vi "NI 5752 Finite Acquisition Multiple Channels (Host).vi"() -> ()   [LabVIEW 2014]
uses:
  <vilib>/rvi/interface/nirviOpenFPGA/nirviOpenFPGA.xnode
  <vilib>/rvi/interface/nirviReadWriteControl/nirviReadWriteControl.xnode
  <vilib>/rvi/interface/nirviCloseFPGA/nirviCloseFPGA.xnode
  <vilib>/rvi/interface/nirviMethod/nirviMethod.xnode
  Program Files (x86)/National Instruments/LabVIEW 2014/examples/FlexRIO/IO Modules/NI 5752/FiniteAcqMultipleChannels/NI 5752 Finite Acquisition Multiple Channels (FPGA).vi
  FPGA Bitfiles/NI5752Fini_PXI-7952R.lvbitx
  <vilib>/LabVIEW Targets/FPGA/FlexRIO/CustomFPGAMethods/79XXR_Method_IOModuleStatusImpl.vi
  NiFpgaLv.dll
  <vilib>/Utility/error.llb/Error Cluster From Error Code.vi
  <vilib>/rvi/errors/niLvFpgaAdjustHostInterfaceError.vi
  <vilib>/FPGAPlugInAG/PXI-7952R/niLvFpga_ReadFifo_PXI-7952R.vi
  <vilib>/rvi/errors/niLvFpgaMergeErrorWithErrorCode.vi
  <vilib>/FPGAPlugInAG/PXI-7952R/niLvFpga_Close_PXI-7952R.vi
  <vilib>/FPGAPlugInAG/PXI-7952R/niLvFpga_Open_PXI-7952R.vi
  <vilib>/userdefined/High Color/nirio_resource_hc.ctl
panel:
  in  "RIO Device":T1="RIO0"
  in  "stop":bool
  in  "ADC D":bool
  in  "ADC C":bool
  in  "ADC B":bool
  in  "ADC A":bool=TRUE
  out "error out":errorcluster
  in  "Tab Control":enum32{"ADC A", " ADC B", "ADC C", "ADC D"}(tab)
  out "ADC A Graph":dbl[][](graph)
  out "ADC B Graph":dbl[][](graph)
  out "ADC C Graph":dbl[][](graph)
  out "ADC D Graph":dbl[][](graph)
  # "ADCs to Acquire"
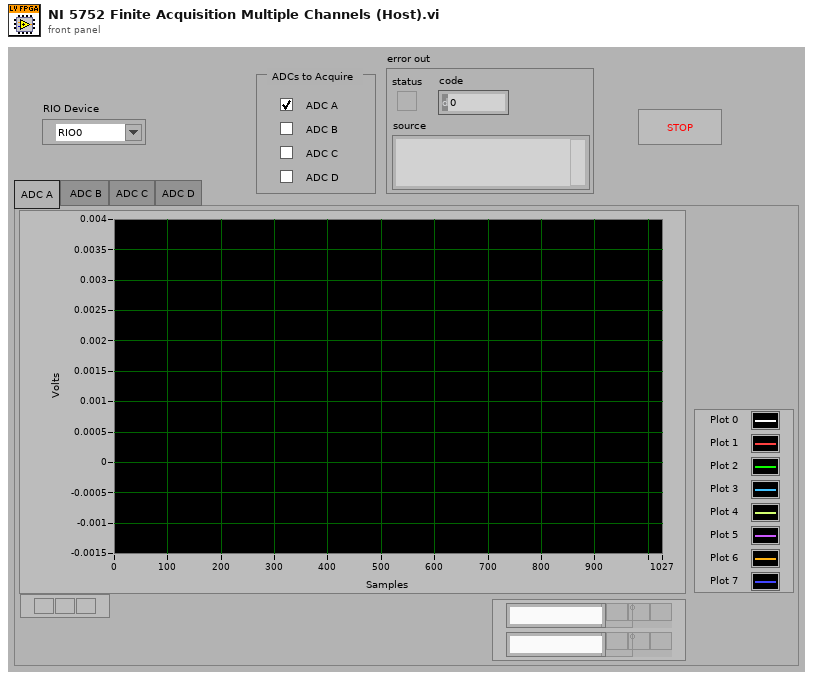
[diagram p1: front panel]
types:
  T1 = typedef "nirio_resource_hc.ctl" = tag
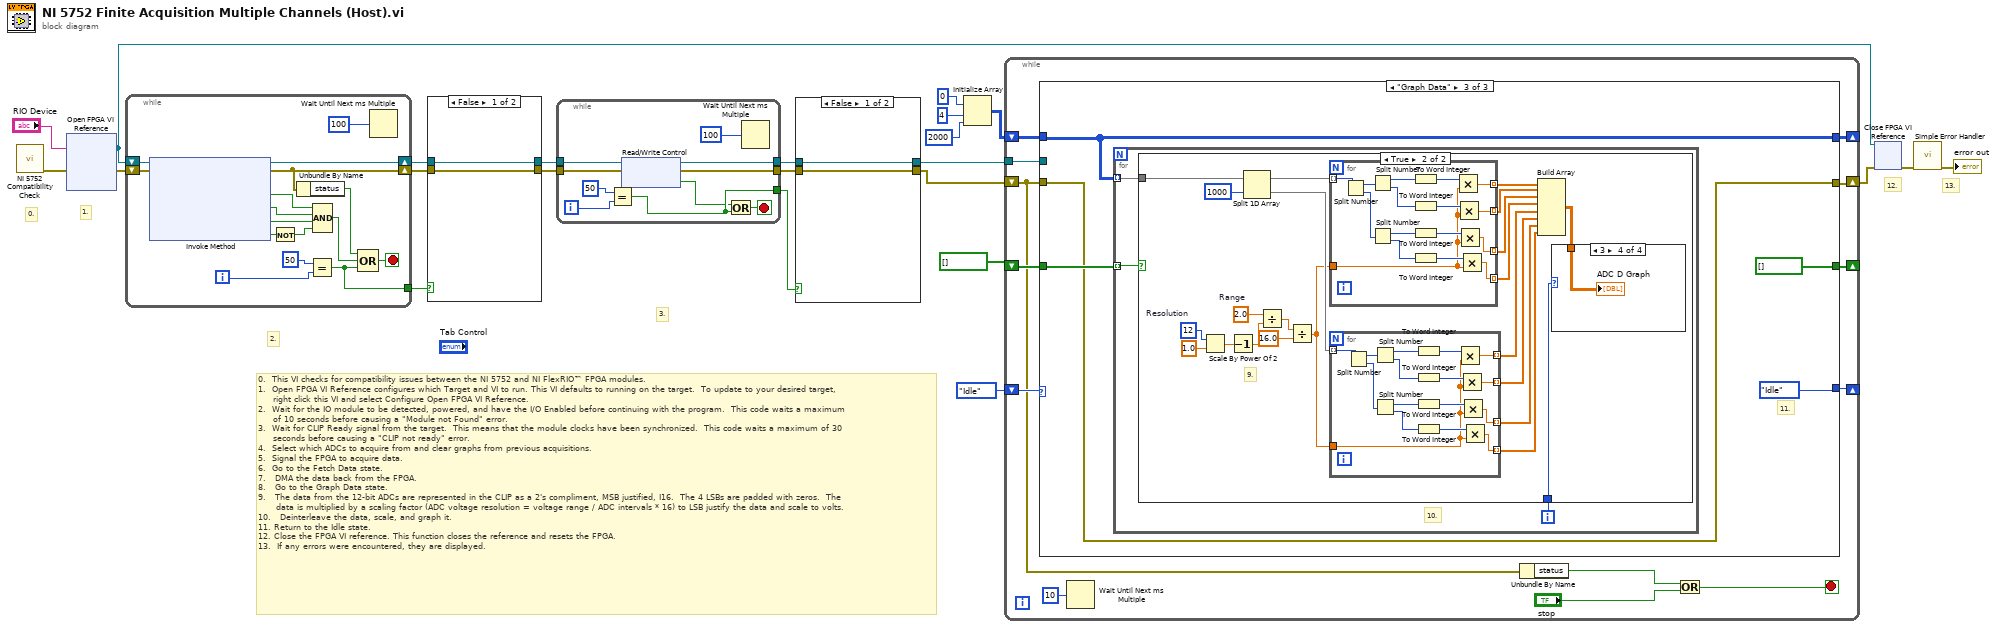
[diagram p0: block diagram]
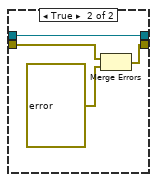
[diagram p2: hidden frame]
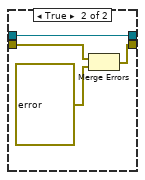
[diagram p3: hidden frame]
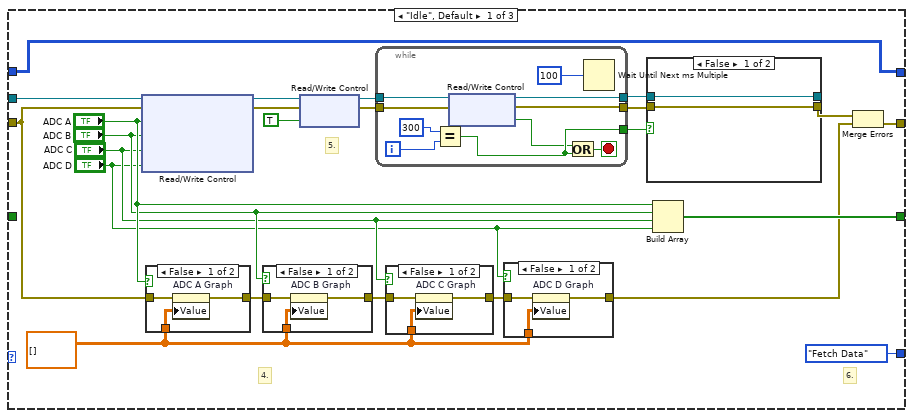
[diagram p4: hidden frame]
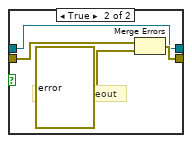
[diagram p5: hidden frame]
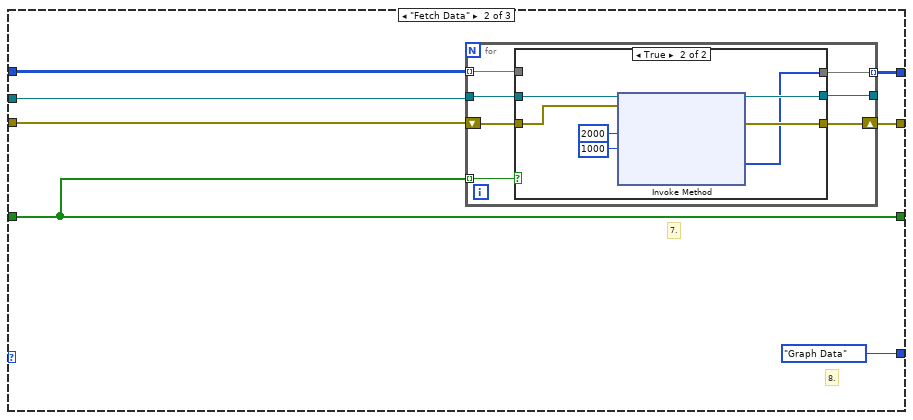
[diagram p10: hidden frame]
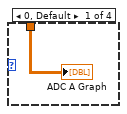
[diagram p13: hidden frame]
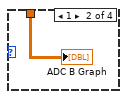
[diagram p14: hidden frame]
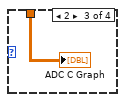
[diagram p15: hidden frame]
diagram:
  # "0."
  # "3."
  # "13."
  # "12."
  # "2."
  # "0.  This VI checks for compatibility issues between the NI 5752 and NI FlexRIO™ FPGA modules. \n1.  Open FPGA VI Reference configures which Target and VI to run. This VI defaults to running on the target.  To update to your desired target, \n     right click this VI and select Configure Open FPGA VI Reference.\n2.  Wait for the IO module to be detected, powered, and have the I/O Enabled before continuing with the program.  This code waits a maximum \n     of 10 seconds before causing a \"Module not Found\" error.\n3.  Wait for CLIP Ready signal from the target.  This means that the module clocks have been synchronized.  This code waits a maximum of 30 \n     seconds before causing a \"CLIP not ready\" error.\n4.  Select which ADCs to acquire from and clear graphs from previous acquisitions.\n5.  Signal the FPGA to acquire data.\n6.  Go to the Fetch Data state.\n7.   DMA the data back from the FPGA.\n8.   Go to the Graph Data state.\n9.   The data from the 12-bit ADCs are represented in the CLIP as a 2's compliment, MSB justified, I16.  The 4 LSBs are padded with zeros.  The \n      data is multiplied by a scaling factor (ADC voltage resolution = voltage range / ADC intervals * 16) to LSB justify the data and scale to volts.\n10.   Deinterleave the data, scale, and graph it.\n11. Return to the Idle state.\n12. Close the FPGA VI reference. This function closes the reference and resets the FPGA.\n13.  If any errors were encountered, they are displayed."
  # "1."
  n1 = call "NI 5752 Compatibility Check.vi"() -> ("error out"=w1:errorcluster)  [unwired: 2 in, 9 out]
  n2 = xnode "Open FPGA VI Reference"("error in"=w1, "resource name"="RIO Device") -> ("FPGA VI Reference Out"=w13:refnum<k20>, "error out"=w14:errorcluster)
  n3 = while {
    shift-right: [w30] -> w12
    shift-left: w14 -> [w38]
    shift-right: [w37] -> w10
    shift-left: w13 -> [w39]
    tunnel: [w26] -> w11
    i -> [w32]
    stop <- w27 stop-if-true
    n4 = xnode "Invoke Method"("FPGA VI Reference In"=w39, "error in"=w38) -> ("FPGA VI Reference Out"=w37:refnum<k20>, "error out"=w30:errorcluster, "IO Module Present?"=w36:bool, "Power Enabled?"=w35:bool, "IO Enabled?"=w34:bool, "IO Module Mismatch?"=w25:bool)
    n5 = Not(x=w25) -> (.not. x?=w24:bool)
    n6 = Unbundle By Name(w30) -> ("status"=w29:bool)
    n7 = Equal?(x=50, y=w32) -> (x = y?=w26:bool)
    n8 = Compound Arithmetic op=AND(w36, w35, w34, w24) -> (w28:bool)
    n9 = Compound Arithmetic op=OR(w29, w28, w26) -> (w27:bool)
    n10 = Wait Until Next ms Multiple(millisecond multiple=u32 100) -> ()  [unwired: 1 out]
  }
  n11 = case shown="False" w11 {
    tunnel: w12 -> [w40 w44]
    tunnel: [w40 w43] -> w8
    tunnel: w10 -> [w41 w42]
    tunnel: [w41 w42] -> w9
    frame False {
    }
    frame True {
      n12 = Merge Errors(w44, errorcluster {"status"=TRUE, "code"=-1, "source"="The IO Module was not present, powered, or the IO were not enabled.  Verify the NI 5752 is securly connected and try again."} ("error in")) -> (w43:errorcluster)
    }
  }
  n13 = while {
    tunnel: w9 -> [w55]
    tunnel: [w51] -> w7
    tunnel: [w50] -> w6
    tunnel: [w48] -> w3
    tunnel: w8 -> [w46]
    i -> [w53]
    stop <- w49 stop-if-true
    n14 = Equal?(x=50, y=w53) -> (x = y?=w48:bool)
    n15 = xnode "Read/Write Control"("FPGA VI Reference In"=w55, "error in"=w46) -> ("FPGA VI Reference Out"=w51:refnum<k20>, "error out"=w50:errorcluster, "Init Done"=w47:bool)
    n16 = Or(x=w47, y=w48) -> (x .or. y?=w49:bool)
    n17 = Wait Until Next ms Multiple(millisecond multiple=u32 100) -> ()  [unwired: 1 out]
  }
  n18 = case shown="False" w3 {
    tunnel: w6 -> [w56 w60]
    tunnel: [w56 w59] -> w4
    tunnel: w7 -> [w57 w58]
    tunnel: [w57 w58] -> w5
    frame False {
    }
    frame True {
      n19 = Merge Errors(w60, errorcluster {"status"=TRUE, "code"=-1, "source"="The IO Module CLIP was not ready. If you are using any external clocks, make sure they are connected and within the supported specifications."} ("error in")) -> (w59:errorcluster)
    }
  }
  n20 = Initialize Array(u64 0, 4 ("dimension size"), 2000 ("dimension size")) -> (w20:u64[][])
  n21 = while {
    shift-right: [w73] -> _
    shift-left: enum16{"Idle", "Graph Data", "Fetch Data"}."Idle" -> [w74]
    tunnel: w5 -> [w66]
    shift-right: [w71] -> _
    shift-left: w20 -> [w72]
    shift-right: [w69] -> _
    shift-left: bool[] [] -> [w68]
    shift-right: [w67] -> w16
    shift-left: w4 -> [w65]
    stop <- w62 stop-if-true
    n22 = case shown="\"Graph Data\"" w74 {
      tunnel: w66 -> [w98 w131 _]
      tunnel: w65 -> [w97 w132 w155]
      tunnel: [w96 w133 w155] -> w67
      tunnel: [enum16{"Idle", "Graph Data", "Fetch Data"}."Fetch Data" enum16{"Idle", "Graph Data", "Fetch Data"}."Graph Data" enum16{"Idle", "Graph Data", "Fetch Data"}."Idle"] -> w73
      tunnel: w72 -> [w94 w136 w156]
      tunnel: [w94 w134 w156] -> w71
      tunnel: [w93 w135 bool[] []] -> w69
      tunnel: w68 -> [_ w135 w157]
      frame "Idle", Default {
        w88 = dbl[][] [] ("ADC A Graph")
        # "6."
        # "5."
        # "4."
        n23 = xnode "Read/Write Control"("FPGA VI Reference In"=w98, "error in"=w97, "ADC A Requested"="ADC A", "ADC B Requested"="ADC B", "ADC C Requested"="ADC C", "ADC D Requested"="ADC D") -> ("FPGA VI Reference Out"=w92:refnum<k20>, "error out"=w89:errorcluster)
        n24 = case shown="False" "ADC A" {
          tunnel: w97 -> [w129 w130]
          tunnel: w88 -> [w128 _]
          tunnel: [w127 w130] -> w87
          frame False {
            n25 = property on="ADC A Graph" class="WFGraph (strict)"(error in=w129, "Value"=w128) -> (error out=w127:errorcluster)  [unwired: 1 in, 1 out]
          }
          frame True {
          }
        }
        n26 = case shown="False" "ADC B" {
          tunnel: w88 -> [w125 _]
          tunnel: w87 -> [w124 w126]
          tunnel: [w123 w126] -> w86
          frame False {
            n27 = property on="ADC B Graph" class="WFGraph (strict)"(error in=w124, "Value"=w125) -> (error out=w123:errorcluster)  [unwired: 1 in, 1 out]
          }
          frame True {
          }
        }
        n28 = xnode "Read/Write Control"("FPGA VI Reference In"=w92, "error in"=w89, "Acquire"=TRUE) -> ("FPGA VI Reference Out"=w79:refnum<k20>, "error out"=w80:errorcluster)
        n29 = while {
          tunnel: w79 -> [w114]
          tunnel: [w110] -> w77
          tunnel: [w109] -> w76
          tunnel: [w107] -> w75
          tunnel: w80 -> [w105]
          i -> [w112]
          stop <- w108 stop-if-true
          n30 = Equal?(x=300, y=w112) -> (x = y?=w107:bool)
          n31 = xnode "Read/Write Control"("FPGA VI Reference In"=w114, "error in"=w105) -> ("FPGA VI Reference Out"=w110:refnum<k20>, "error out"=w109:errorcluster, "Init Done"=w106:bool)
          n32 = Or(x=w106, y=w107) -> (x .or. y?=w108:bool)
          n33 = Wait Until Next ms Multiple(millisecond multiple=u32 100) -> ()  [unwired: 1 out]
        }
        n34 = case shown="False" "ADC C" {
          tunnel: w88 -> [w121 _]
          tunnel: w86 -> [w120 w122]
          tunnel: [w119 w122] -> w85
          frame False {
            n35 = property on="ADC C Graph" class="WFGraph (strict)"(error in=w120, "Value"=w121) -> (error out=w119:errorcluster)  [unwired: 1 in, 1 out]
          }
          frame True {
          }
        }
        n36 = case shown="False" "ADC D" {
          tunnel: [w117 w118] -> w91
          tunnel: w88 -> [w116 _]
          tunnel: w85 -> [w115 w118]
          frame False {
            n37 = property on="ADC D Graph" class="WFGraph (strict)"(error in=w115, "Value"=w116) -> (error out=w117:errorcluster)  [unwired: 1 in, 1 out]
          }
          frame True {
          }
        }
        n38 = case shown="False" w75 {
          tunnel: [w100 w102] -> _
          tunnel: w77 -> [w100 w102]
          tunnel: w76 -> [w99 w101]
          tunnel: [w99 w104] -> w78
          frame False {
          }
          frame True {
            # "InitDone timeout"
            n39 = Merge Errors(w101, errorcluster {"status"=TRUE, "code"=-1, "source"="The IO Module CLIP was not ready. If you are using any external clocks, make sure they are connected and within the supported specifications."} ("error in")) -> (w104:errorcluster)
          }
        }
        n40 = Build Array("ADC A", "ADC B", "ADC C", "ADC D") -> (w93:bool[])
        n41 = Merge Errors(w78, w91) -> (w96:errorcluster)
      }
      frame "Fetch Data" {
        # "8."
        # "7."
        n42 = for {
          tunnel: w131 -> [w144]
          tunnel: w136 -> [w140] mode=indexing
          tunnel: [w143] -> w134 mode=indexing
          tunnel: w135 -> [w141] mode=indexing
          shift-right: [w138] -> w133
          shift-left: w132 -> [w142]
          tunnel: [w139] -> _
          n43 = case shown="True" w141 {
            tunnel: w144 -> [w145 w154]
            tunnel: [w147 w148] -> w143
            tunnel: w142 -> [w146 w153]
            tunnel: [w146 w152] -> w138
            tunnel: w140 -> [w147 _]
            tunnel: [w145 w151] -> w139
            frame False {
            }
            frame True {
              n44 = xnode "Invoke Method"("FPGA VI Reference In"=w154, "error in"=w153, "Number of Elements"=u32 2000, "Timeout (ms)"=1000) -> ("FPGA VI Reference Out"=w151:refnum<k20>, "error out"=w152:errorcluster, "Data"=w148:u64[])  [unwired: 1 out]
            }
          }
        }
      }
      frame "Graph Data" {
        # "11."
        n45 = for {
          tunnel: w157 -> [w161] mode=indexing
          tunnel: w156 -> [w162] mode=indexing
          i -> [w160]
          # "10."
          n46 = case shown="True" w161 {
            tunnel: w162 -> [_ w180]
            tunnel: w160 -> [_ w171]
            frame False {
            }
            frame True {
              w168 = 12  # Resolution
              w166 = 2.0  # Range
              # "9."
              n47 = Scale By Power Of 2(n=w168, x=1.0) -> (x*2^n=w169:dbl)
              n48 = Decrement(x=w169) -> (x-1=w170:dbl)
              n49 = Split 1D Array(array=w180, index=1000) -> (first subarray=w178:u64[], second subarray=w177:u64[])
              n50 = Divide(x=w166, y=w170) -> (x/y=w165:dbl)
              n51 = Divide(x=w165, y=16.0) -> (x/y=w164:dbl)
              n52 = for {
                tunnel: w178 -> [w216] mode=indexing
                tunnel: [w205] -> w184 mode=indexing
                tunnel: [w204] -> w183 mode=indexing
                tunnel: [w203] -> w182 mode=indexing
                tunnel: [w202] -> w181 mode=indexing
                tunnel: w164 -> [w201]
                n53 = Split Number(x=w216) -> (hi(x)=w215:u32, lo(x)=w214:u32)
                n54 = Split Number(x=w215) -> (hi(x)=w213:u16, lo(x)=w210:u16)
                n55 = Split Number(x=w214) -> (hi(x)=w207:u16, lo(x)=w206:u16)
                n56 = To Word Integer(number=w213) -> (16bit integer=w212:i16)
                n57 = To Word Integer(number=w210) -> (16bit integer=w211:i16)
                n58 = To Word Integer(number=w207) -> (16bit integer=w209:i16)
                n59 = To Word Integer(number=w206) -> (16bit integer=w208:i16)
                n60 = Multiply(x=w212, y=w201) -> (x*y=w205:dbl)
                n61 = Multiply(x=w211, y=w201) -> (x*y=w204:dbl)
                n62 = Multiply(x=w209, y=w201) -> (x*y=w203:dbl)
                n63 = Multiply(x=w208, y=w201) -> (x*y=w202:dbl)
              }
              n64 = for {
                tunnel: w177 -> [w200] mode=indexing
                tunnel: [w189] -> w176 mode=indexing
                tunnel: [w188] -> w175 mode=indexing
                tunnel: [w187] -> w174 mode=indexing
                tunnel: [w186] -> w173 mode=indexing
                tunnel: w164 -> [w185]
                n65 = Split Number(x=w200) -> (hi(x)=w199:u32, lo(x)=w198:u32)
                n66 = Split Number(x=w199) -> (hi(x)=w197:u16, lo(x)=w194:u16)
                n67 = Split Number(x=w198) -> (hi(x)=w191:u16, lo(x)=w190:u16)
                n68 = To Word Integer(number=w197) -> (16bit integer=w196:i16)
                n69 = To Word Integer(number=w194) -> (16bit integer=w195:i16)
                n70 = To Word Integer(number=w191) -> (16bit integer=w193:i16)
                n71 = To Word Integer(number=w190) -> (16bit integer=w192:i16)
                n72 = Multiply(x=w196, y=w185) -> (x*y=w189:dbl)
                n73 = Multiply(x=w195, y=w185) -> (x*y=w188:dbl)
                n74 = Multiply(x=w193, y=w185) -> (x*y=w187:dbl)
                n75 = Multiply(x=w192, y=w185) -> (x*y=w186:dbl)
              }
              n76 = Build Array(w184, w183, w182, w181, w176, w175, w174, w173) -> (w172:dbl[][])
              n77 = case shown="3" w171 {
                tunnel: w172 -> [w217 w218 w219 w220]
                frame 0, Default {
                  "ADC A Graph" <- w217
                }
                frame 1 {
                  "ADC B Graph" <- w218
                }
                frame 2 {
                  "ADC C Graph" <- w219
                }
                frame 3 {
                  "ADC D Graph" <- w220
                }
              }
            }
          }
        }
      }
    }
    n78 = Wait Until Next ms Multiple(millisecond multiple=u32 10) -> ()  [unwired: 1 out]
    n79 = Unbundle By Name(w65) -> ("status"=w64:bool)
    n80 = Or(x=w64, y="stop") -> (x .or. y?=w62:bool)
  }
  n81 = xnode "Close FPGA VI Reference"("FPGA VI Reference In"=w13, "error in"=w16) -> ("error out"=w17:errorcluster)
  n82 = call <vilib>:"Simple Error Handler.vi"("error in (no error)"=w17) -> ("error out"=→"error out":errorcluster)  [unwired: 1 in, 7 out]
